vi "bubble.vi"() -> ()   [LabVIEW 2019]
uses:
  <vilib>/myRIO/Instrument Drivers/Onboard Devices/Accelerometer/typedefs/Accelerometer Reference.ctl
  <vilib>/myRIO/Common/Instrument Driver Framework/Utilities/typedefs/myRIO Generic Hardware Reference.ctl
  <vilib>/myRIO/Common/Instrument Driver Framework/Utilities/typedefs/Hardware Version Enum.ctl
  <vilib>/myRIO/Common/Instrument Driver Framework/Utilities/typedefs/myRIO v1.0 Reference.ctl
  <vilib>/myRIO/Common/Instrument Driver Framework/Utilities/typedefs/Generic FPGA Reference.ctl
  <vilib>/myRIO/Common/Instrument Driver Framework/myRIO v1.0/Accelerometer/typedefs/Accelerometer Channels List.ctl
  <vilib>/myRIO/Common/Instrument Driver Framework/myRIO v1.0/Accelerometer/typedefs/Accelerometer Channels Enum.ctl
  <vilib>/userDefined/High Color/nirio_resource_hc.ctl
  <vilib>/myRIO/Instrument Drivers/Onboard IO/DIO/typedefs/DIO Reference.ctl
  <vilib>/myRIO/Common/Instrument Driver Framework/myRIO v1.0/DIO/typedefs/DIO Channels List.ctl
  <vilib>/myRIO/Common/Instrument Driver Framework/myRIO v1.0/DIO/typedefs/DIO Channels Enum.ctl
  <vilib>/myRIO/Common/Instrument Driver Framework/Utilities/vis/Is FPGA Ref Available.vi
  <vilib>/myRIO/Common/Instrument Driver Framework/myRIO v1.0/Accelerometer/vis/myRIO v1.1 Open Accelerometer.vi
  <vilib>/myRIO/Instrument Drivers/Onboard Devices/Accelerometer/vis/Read.vi
  <vilib>/myRIO/Common/Instrument Driver Framework/myRIO v1.0/DIO/vis/myRIO v1.1 Open DIO.vi
  <vilib>/myRIO/Instrument Drivers/Onboard IO/DIO/vis/Read.vi
  <vilib>/myRIO/Instrument Drivers/Onboard IO/DIO/vis/Write.vi
  <vilib>/myRIO/Common/Instrument Driver Framework/Utilities/vis/Validate Channels.vi
  <vilib>/myRIO/Common/Instrument Driver Framework/myRIO v1.0/Accelerometer/vis/myRIO v1.0 Reserve Accelerometer.vi
  <vilib>/myRIO/Common/Instrument Driver Framework/myRIO v1.0/DIO/vis/myRIO v1.0 Reserve DIO.vi
  <vilib>/myRIO/Common/Instrument Driver Framework/myRIO v1.0/Resource Manager/vis/myRIO v1.0 Reserve Channel List.vi
  <vilib>/myRIO/Common/Instrument Driver Framework/myRIO v1.0/Accelerometer/vis/myRIO v1.0 Build MUX Configuration Accelerometer.vi
  <vilib>/myRIO/Common/Instrument Driver Framework/myRIO v1.0/DIO/vis/myRIO v1.0 Build MUX Configuration DIO.vi
  <vilib>/myRIO/Common/Instrument Driver Framework/myRIO v1.0/Resource Manager/vis/myRIO v1.0 Reserve Channel.vi
  <vilib>/myRIO/Common/Instrument Driver Framework/myRIO v1.0/Resource Manager/vis/myRIO v1.0 Unreserve Channel.vi
  <vilib>/myRIO/Common/Instrument Driver Framework/myRIO v1.0/Resource Manager/vis/myRIO v1.0 Create Configuration List.vi
  <vilib>/myRIO/Common/Instrument Driver Framework/myRIO v1.0/Resource Manager/vis/myRIO v1.0 Build Mutex Name.vi
  <vilib>/Utility/VariantDataType/GetNumericInfo.vi
  <vilib>/Utility/error.llb/Error Cluster From Error Code.vi
  <vilib>/myRIO/Common/Instrument Driver Framework/myRIO v1.0/myRIO v1.1 Open.vi
  <vilib>/myRIO/Common/Instrument Driver Framework/myRIO v1.0/Accelerometer/vis/myRIO v1.0 Get Scaling Constant Accelerometer.vi
  <vilib>/myRIO/Common/Instrument Driver Framework/Utilities/vis/IO Manager.vi
  <vilib>/myRIO/Common/Instrument Driver Framework/Utilities/vis/Configuration Manager.vi
  <vilib>/myRIO/Common/Instrument Driver Framework/myRIO v1.0/myRIO v1.0 Close.vi
  <vilib>/myRIO/Common/Instrument Driver Framework/myRIO v1.0/Accelerometer/vis/myRIO v1.0 Read Accelerometer.vi
  <vilib>/myRIO/Common/Instrument Driver Framework/myRIO v1.0/Resource Manager/vis/myRIO v1.0 Configure IO.vi
  <vilib>/myRIO/Common/Instrument Driver Framework/myRIO v1.0/DIO/vis/myRIO v1.0 Read DIO.vi
  <vilib>/myRIO/Common/Instrument Driver Framework/myRIO v1.0/DIO/vis/myRIO v1.0 Write DIO.vi
  <vilib>/myRIO/Express VI/Onboard Devices/Accelerometer/Accelerometer Express VI.xnode
  <vilib>/myRIO/Instrument Drivers/Onboard Devices/Accelerometer/vis/myRIO Accelerometer Open.xnode
  <vilib>/myRIO/Express VI/Onboard Devices/Button/Button Express VI.xnode
  <vilib>/myRIO/Instrument Drivers/Onboard IO/DIO/vis/myRIO DIO Open.xnode
  <vilib>/myRIO/Express VI/Onboard Devices/LED/LED Express VI.xnode
  <vilib>/myRIO/Instrument Drivers/Onboard Devices/Accelerometer/Accelerometer.lvlib
  <vilib>/myRIO/Instrument Drivers/Onboard IO/DIO/DIO.lvlib
panel:
  in  "stop":bool
  out "error out":errorcluster
  out "Angle value":dbl
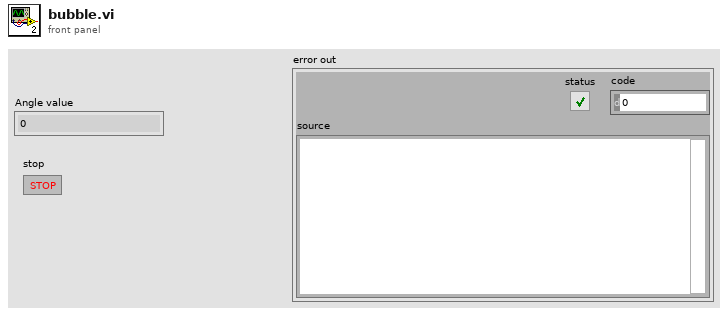
[diagram p1: front panel]
types:
  T1 = enum16{"open", "replace", "create", "open or create", "replace or create", "replace or create with confirmation"}
  T2 = typedef "DIO.lvlib/DIO Reference.ctl" = cluster{"myRIO Reference":T3, "DIO Channels List":T7}
  T3 = typedef "myRIO Generic Hardware Reference.ctl" = cluster{"myRIO Model":T4, "myRIO Hardware Reference":T5}
  T4 = typedef "Hardware Version Enum.ctl" = enum16{"Unknown", "myRIO-1900", "myRIO-1950", "roboRIO", "NI ELVIS RIO CM", "ELVIS III"}
  T5 = typedef "myRIO v1.0 Reference.ctl" = cluster{"Generic FPGA Reference":T6, "Allow multiple opens":bool}
  T6 = typedef "Generic FPGA Reference.ctl" = refnum<k20>
  T7 = typedef "DIO Channels List.ctl" = T8[]
  T8 = typedef "DIO Channels Enum.ctl" = enum16{"Not Connected", "C/DIO0", "C/DIO1", "C/DIO2", "C/DIO3", "C/DIO4", "C/DIO5", "C/DIO6", "C/DIO7", "A/DIO0", "A/DIO1", "A/DIO2", "A/DIO3", "A/DIO4", "A/DIO5", "A/DIO6", "A/DIO7", "A/DIO8", "A/DIO9", "A/DIO10", "A/DIO11", "A/DIO12", "A/DIO13", "A/DIO14", "A/DIO15", "A/DIO16", "A/DIO17", "A/DIO18", "A/DIO19", "B/DIO0", "B/DIO1", "B/DIO2", "B/DIO3", "B/DIO4", "B/DIO5", "B/DIO6", "B/DIO7", "B/DIO8", "B/DIO9", "B/DIO10", "B/DIO11", "B/DIO12", "B/DIO13", "B/DIO14", "B/DIO15", "B/DIO16", "B/DIO17", "B/DIO18", "B/DIO19", "LED0", "LED1", "LED2", "LED3", "Button0", "DIO/DIO0", "DIO/DIO1", "DIO/DIO2", "DIO/DIO3", "DIO/DIO4", "DIO/DIO5", "DIO/DIO6", "DIO/DIO7", "DIO/DIO8", "DIO/DIO9", "SPI/CS0", "SPI/CS1", "SPI/CS2", "SPI/CS3", "LED RADIO (Green)", "LED RADIO (Red)", "LED COMM (Green)", "LED COMM (Red)", "LED MODE (Green)", "LED MODE (Red)"}
  T9 = typedef "nirio_resource_hc.ctl" = tag
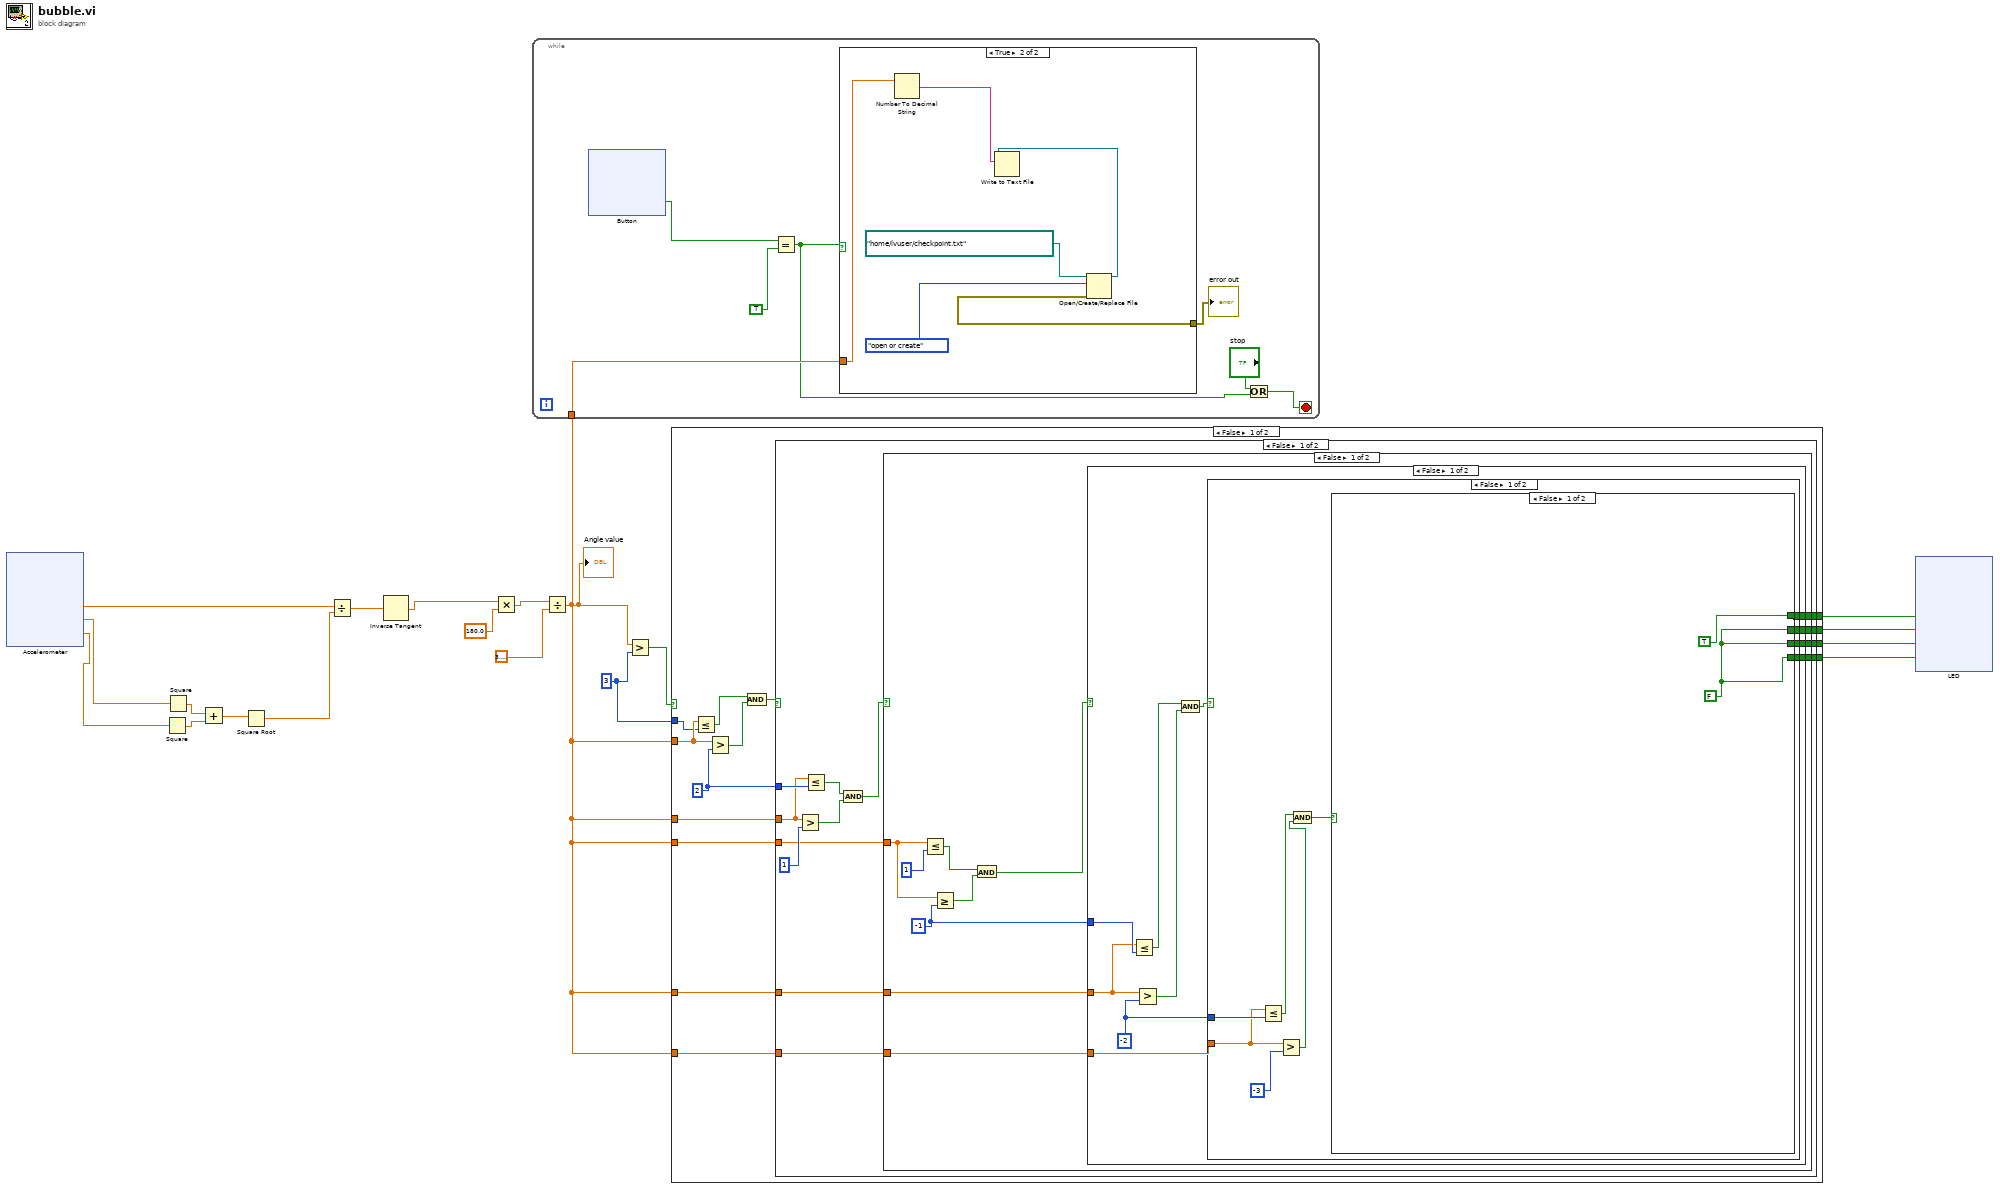
[diagram p0: block diagram]
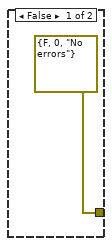
[diagram p2: hidden frame]
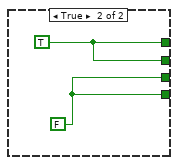
[diagram p3: hidden frame]
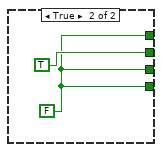
[diagram p4: hidden frame]
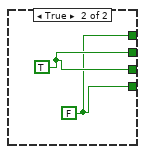
[diagram p5: hidden frame]
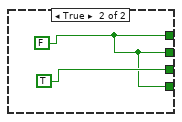
[diagram p6: hidden frame]
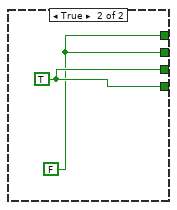
[diagram p7: hidden frame]
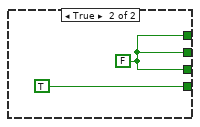
[diagram p8: hidden frame]
diagram:
  w5 = 3
  n1 = xnode "Accelerometer"() -> ("X-Axis"=w9:dbl, "Y-Axis"=w14:dbl, "Z-Axis"=w13:dbl)  [unwired: 1 in, 1 out]
  n2 = Square(x=w13) -> (x^2=w12:dbl)
  n3 = Square(x=w14) -> (x^2=w11:dbl)
  n4 = Add(x=w11, y=w12) -> (x+y=w10:dbl)
  n5 = Square Root(x=w10) -> (sqrt(x)=w8:dbl)
  n6 = Divide(x=w9, y=w8) -> (x/y=w7:dbl)
  n7 = Inverse Tangent(1:w7) -> (0:w6:dbl)
  n8 = Multiply(x=w6, y=180.0) -> (x*y=w18:dbl)
  n9 = Divide(x=w18, y=3.141592653589793) -> (x/y=w15:dbl)
  "Angle value" <- w15
  n10 = while {
    tunnel: w15 -> [w24]
    stop <- w20 stop-if-true
    n11 = xnode "Button"() -> ("Value"=w26:bool)  [unwired: 1 in, 1 out]
    n12 = Equal?(x=w26, y=TRUE) -> (x = y?=w21:bool)
    n13 = case shown="True" w21 {
      tunnel: w24 -> [_ w33]
      tunnel: [errorcluster {"status"=FALSE, "code"=0, "source"="No errors"} ("error out") w31] -> w23
      frame False {
      }
      frame True {
        n14 = Number To Decimal String(number=w33) -> (decimal integer string=w29:string)  [unwired: 1 in]
        n15 = Open/Create/Replace File(file path (use dialog)=path "/home/lvuser/checkpoint.txt", operation (0:open)=T1."open or create") -> (refnum out=w28:refnum<file>, error out=w31:errorcluster)  [unwired: 4 in, 1 out]
        n16 = Write to Text File(file (use dialog)=w28, text=w29) -> ()  [unwired: 2 in, 3 out]
      }
    }
    "error out" <- w23
    n17 = Or(x="stop", y=w21) -> (x .or. y?=w20:bool)
  }
  n18 = Greater?(x=w15, y=w5) -> (0:w16:bool)
  n19 = case shown="False" w16 {
    tunnel: w15 -> [w74 _]
    tunnel: w15 -> [w82 _]
    tunnel: w15 -> [w81 _]
    tunnel: w15 -> [w80 _]
    tunnel: w15 -> [w79 _]
    tunnel: w5 -> [w73 _]
    tunnel: [w69 TRUE] -> w4
    tunnel: [w72 w141] -> w3
    tunnel: [w71 w141] -> w2
    tunnel: [w70 w141] -> w1
    frame False {
      w75 = 2
      n20 = Less Or Equal?(x=w74, y=w73) -> (x <= y?=w78:bool)
      n21 = Greater?(x=w74, y=w75) -> (0:w77:bool)
      n22 = And(x=w78, y=w77) -> (x .and. y?=w76:bool)
      n23 = case shown="False" w76 {
        tunnel: w82 -> [w90 _]
        tunnel: w81 -> [w94 _]
        tunnel: w80 -> [w93 _]
        tunnel: w79 -> [w92 _]
        tunnel: w75 -> [w91 _]
        tunnel: [w86 w140] -> w72
        tunnel: [w84 w139] -> w71
        tunnel: [w85 w139] -> w70
        tunnel: [w83 w140] -> w69
        frame False {
          n24 = Greater?(x=w90, y=1) -> (0:w87:bool)
          n25 = Less Or Equal?(x=w90, y=w91) -> (x <= y?=w88:bool)
          n26 = And(x=w88, y=w87) -> (x .and. y?=w89:bool)
          n27 = case shown="False" w89 {
            tunnel: w94 -> [w106 _]
            tunnel: w93 -> [w102 _]
            tunnel: w92 -> [w101 _]
            tunnel: [w96 TRUE] -> w86
            tunnel: [w99 w137] -> w85
            tunnel: [w97 w137] -> w84
            tunnel: [w98 w137] -> w83
            frame False {
              w100 = -1
              n28 = Less Or Equal?(x=w106, y=1) -> (x <= y?=w105:bool)
              n29 = Greater Or Equal?(x=w106, y=w100) -> (x >= y?=w104:bool)
              n30 = And(x=w105, y=w104) -> (x .and. y?=w103:bool)
              n31 = case shown="False" w103 {
                tunnel: w102 -> [w116 _]
                tunnel: w101 -> [w118 _]
                tunnel: w100 -> [w117 _]
                tunnel: [w110 w135] -> w99
                tunnel: [w108 w135] -> w98
                tunnel: [w111 w136] -> w97
                tunnel: [w109 w136] -> w96
                frame False {
                  w112 = -2
                  n32 = Less Or Equal?(x=w116, y=w117) -> (x <= y?=w115:bool)
                  n33 = Greater?(x=w116, y=w112) -> (0:w114:bool)
                  n34 = And(x=w115, y=w114) -> (x .and. y?=w113:bool)
                  n35 = case shown="False" w113 {
                    tunnel: w118 -> [w126 _]
                    tunnel: w112 -> [w127 _]
                    tunnel: [w121 TRUE] -> w111
                    tunnel: [w122 w133] -> w110
                    tunnel: [w120 w133] -> w109
                    tunnel: [w119 w133] -> w108
                    frame False {
                      n36 = Less Or Equal?(x=w126, y=w127) -> (x <= y?=w123:bool)
                      n37 = Greater?(x=w126, y=-3) -> (0:w124:bool)
                      n38 = And(x=w123, y=w124) -> (x .and. y?=w125:bool)
                      n39 = case shown="False" w125 {
                        tunnel: [TRUE w132] -> w122
                        tunnel: [w129 w132] -> w121
                        tunnel: [w129 w131] -> w120
                        tunnel: [w129 w131] -> w119
                        frame False {
                          w129 = FALSE
                        }
                        frame True {
                          w131 = FALSE
                          w132 = TRUE
                        }
                      }
                    }
                    frame True {
                      w133 = FALSE
                    }
                  }
                }
                frame True {
                  w135 = FALSE
                  w136 = TRUE
                }
              }
            }
            frame True {
              w137 = FALSE
            }
          }
        }
        frame True {
          w140 = TRUE
          w139 = FALSE
        }
      }
    }
    frame True {
      w141 = FALSE
    }
  }
  n40 = xnode "LED"("LED0"=w1, "LED1"=w2, "LED2"=w3, "LED3"=w4) -> ()  [unwired: 1 in, 1 out]
